vi "ABB Test Locked Rotor.vi"() -> ()   [LabVIEW 2017]
uses:
  Temp error msg.ctl
  ABB global.vi
panel:
  in  "Temp error":T1="Error: Temperature measurement "
  out "Auto Readings":cluster{"%":dbl[], "Recorded":bool[]}
  in  "Simulate I":dbl(slide)
  out "Readings":string[][](table)
  out "In Range?":bool[](array[boolean])
  out "saved Readings":dbl[][](array[numeric])
  out "% rated current":dbl format="%.1f"
  out "Rated Current":dbl
  out "Serial number":string
  out "W.O number":string
  out "Power":string[][](table)
  out "Current & Voltage":string[][](table)
  out "Norma 5000 Error":string
  in  "Record":bool
  out "Readings":string[][](table)
  in  "View":enum16{"Graph", "Readings"}(ring)
  out "Number readings":i32
  out "Status":enum16{"Stopped", "Running"}(ring)
  out "Timedate":string
  in  "End test":bool
  in  "Start":bool
  in  "Read Mode":enum16{"Auto", "Manual"}(ring)
  in  "Exit":bool
  out "Current vs Voltage":T2(graph)
  # "Locked Rotor Test"
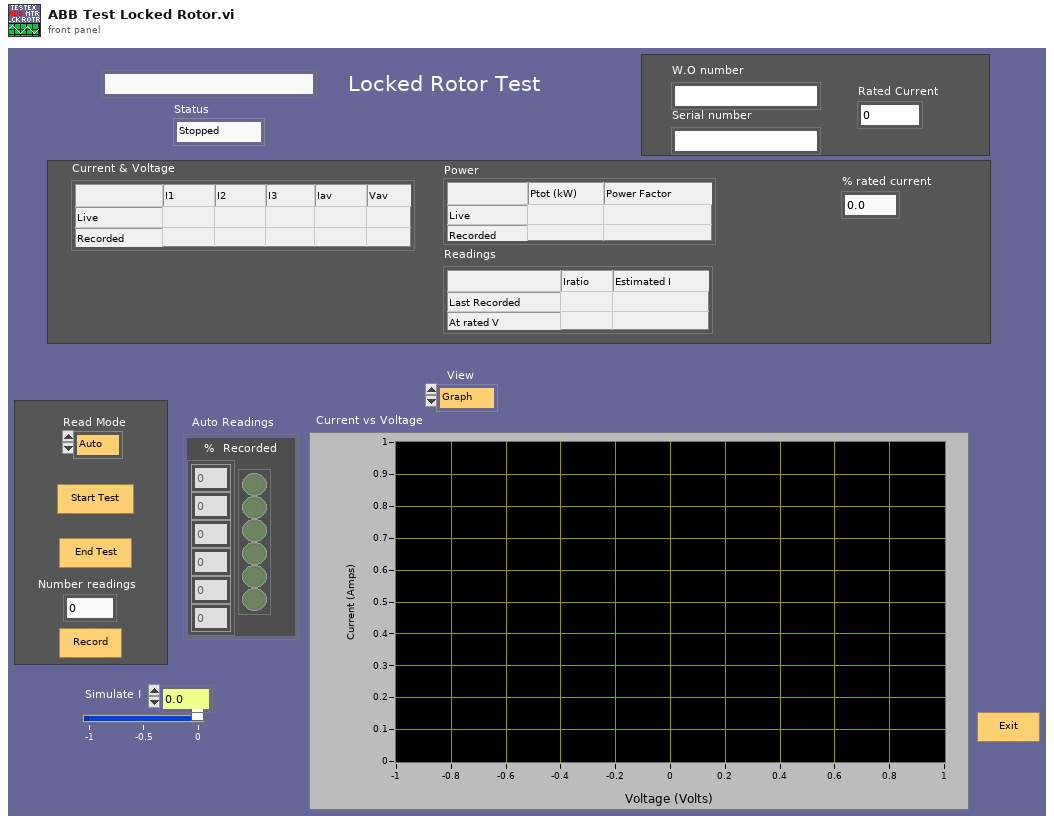
[diagram p1: front panel]
types:
  T1 = typedef "Temp error msg.ctl" = string
  T2 = cluster{"Sorted 2D Array":dbl[], "Sorted 2D Array":dbl[]}
  T3 = cluster{"Voltage":dbl, "Power":dbl, "Current":dbl, "PF":dbl}
  T4 = cluster{"VT Primary":dbl, "VT Secondary":dbl, "CT  Primary":dbl, "CT Secondary":dbl, "Current Shunt":enum16{"Internal", "External"}, "Avg interval":dbl}
  T5 = cluster{"VT Primary":dbl, "VT Secondary":dbl, "CT  Primary":dbl, "CT Secondary":dbl, "Current Shunt":enum16{"Internal", "External"}, "Averaging interval (secs)":dbl}
  T6 = cluster{"Visa sesssion":refnum<visa-resource-name>, "error":errorcluster}
  T7 = cluster{"Simulate Norma":bool, "Norma 5000 Address":u8, "WebDaq IP Address":string, "Simulate cDAQ":bool}
  T8 = cluster{"Number Values":i32, "Tolerance":dbl, "Value (ratio) ":dbl[], "Hold time (sec)":dbl}
  T9 = cluster{"V":dbl, "A":dbl, "W":dbl, "VA":dbl, "VAr":dbl, "Pf":dbl}
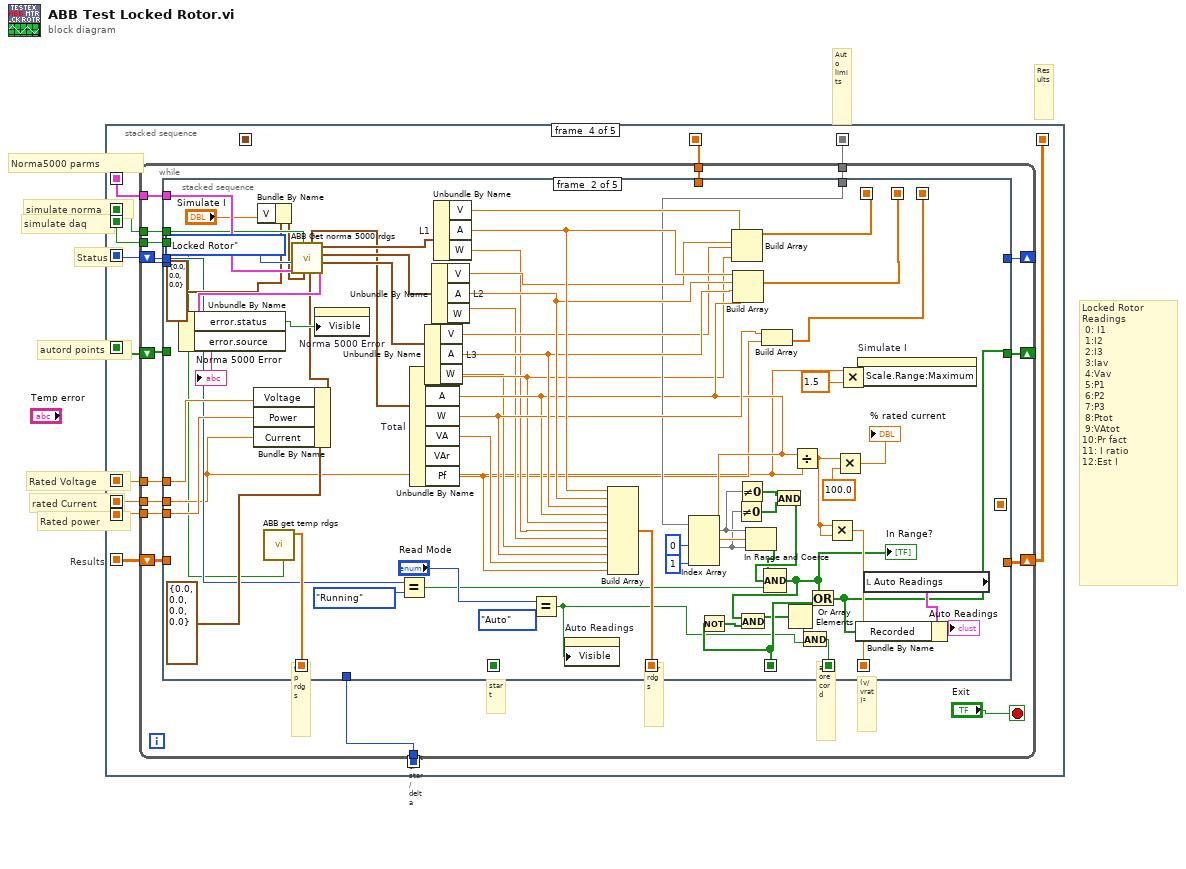
[diagram p0: block diagram]
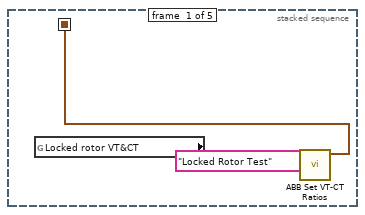
[diagram p2: hidden frame]
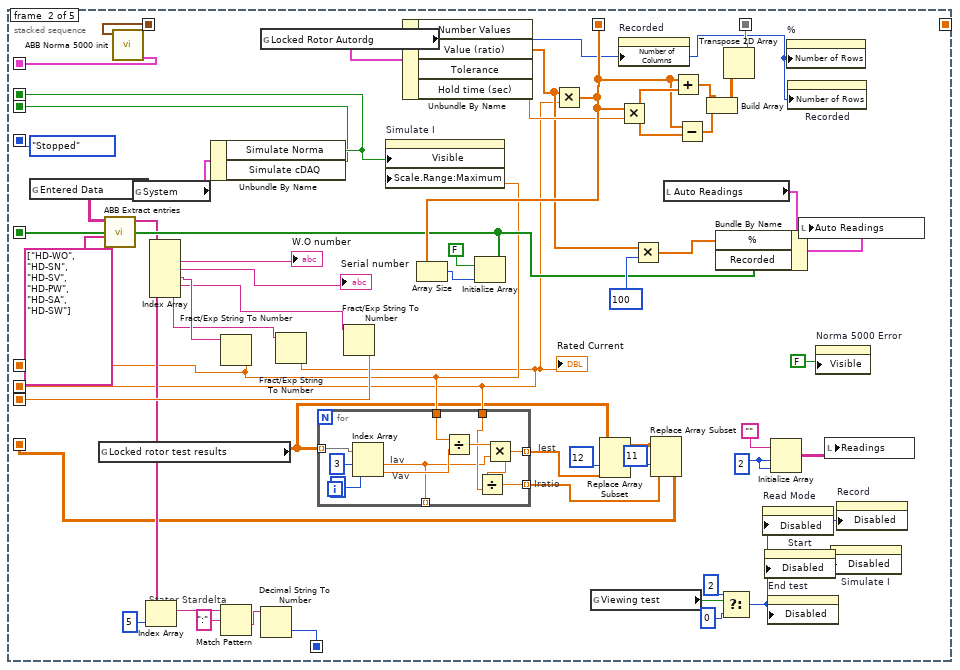
[diagram p3: hidden frame]
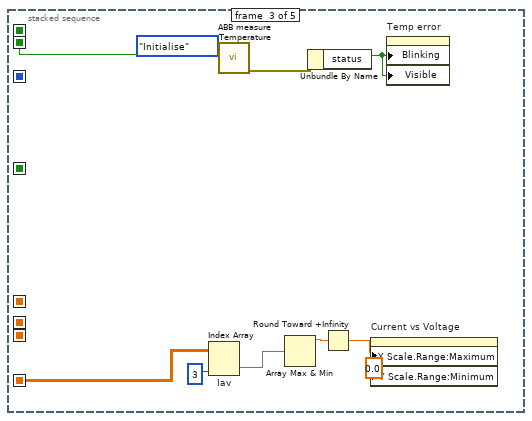
[diagram p4: hidden frame]
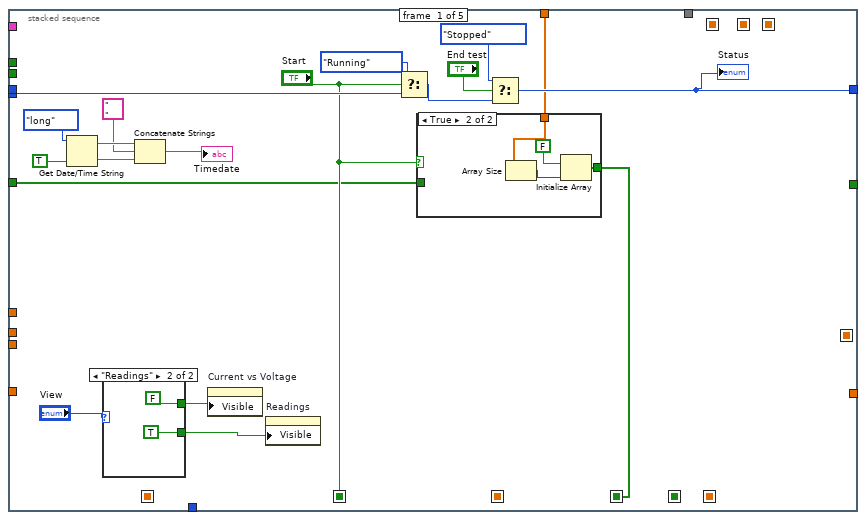
[diagram p5: hidden frame]
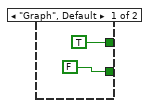
[diagram p7: hidden frame]
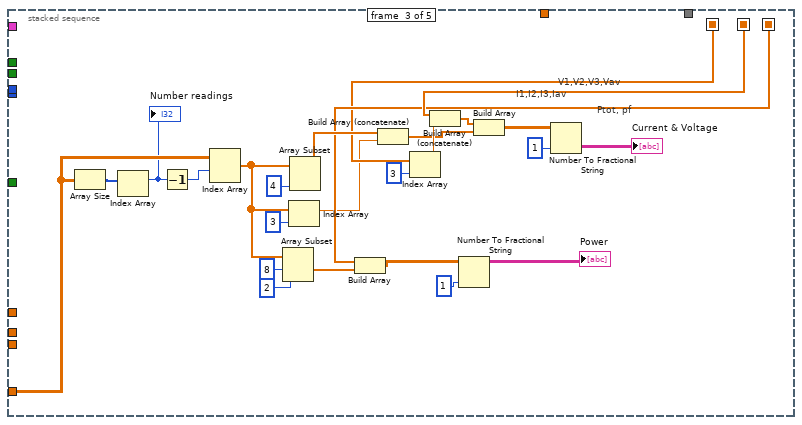
[diagram p8: hidden frame]
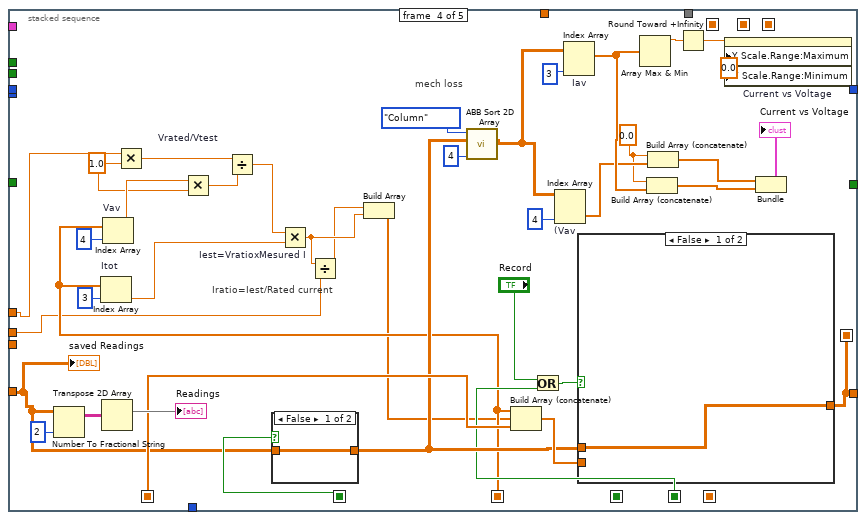
[diagram p9: hidden frame]
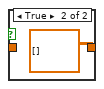
[diagram p10: hidden frame]
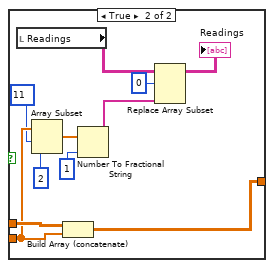
[diagram p11: hidden frame]
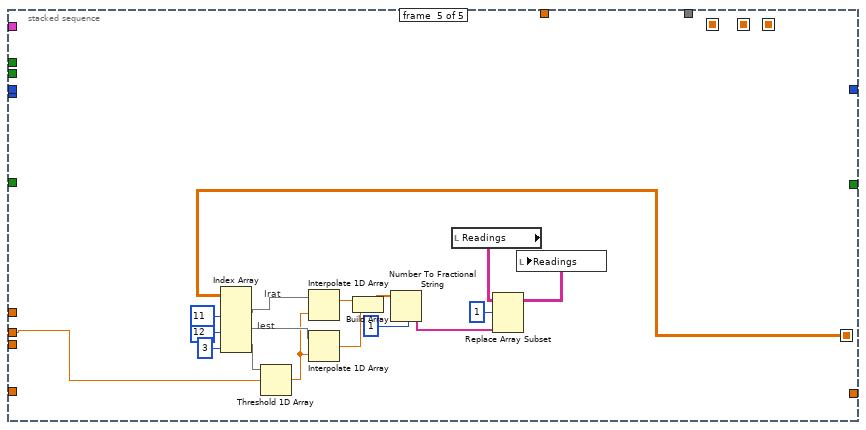
[diagram p12: hidden frame]
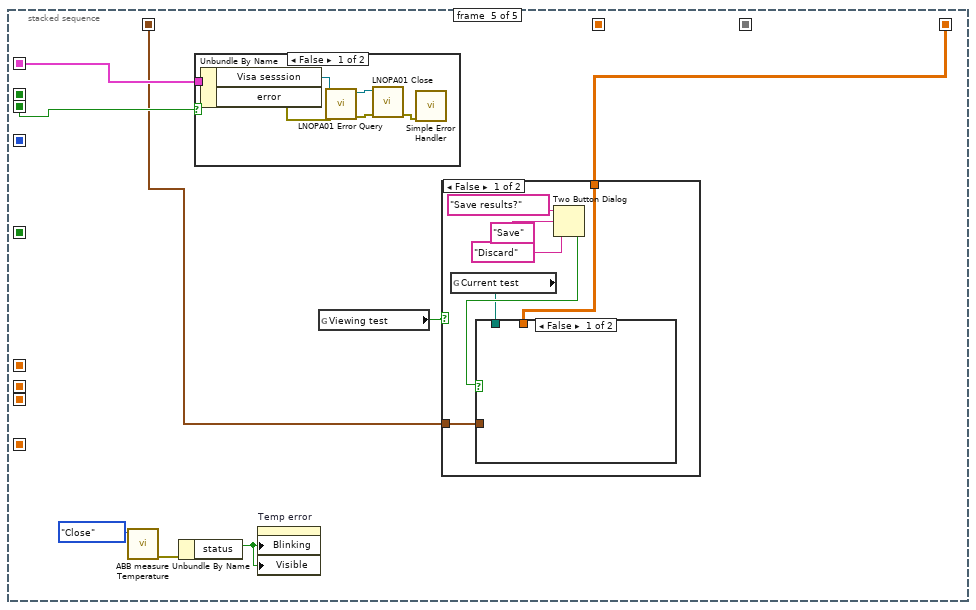
[diagram p13: hidden frame]
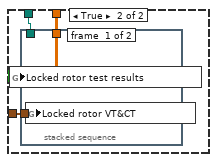
[diagram p14: hidden frame]
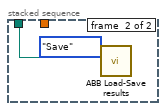
[diagram p15: hidden frame]
diagram:
  # "Results"
  # "stator star/delta"
  # "simulate daq"
  # "Results"
  # "Rated power"
  # "Rated Voltage"
  # "Locked Rotor\nReadings\n 0: I1\n 1:I2\n 2:I3\n 3:Iav\n 4:Vav\n 5:P1\n 6:P2\n 7:P3\n 8:Ptot\n 9:VAtot\n10:Pr fact\n11: I ratio\n12:Est I"
  # "autord points"
  # "Auto limits"
  # "rated Current"
  # "simulate norma"
  # "Norma5000 parms"
  # "Status"
  n1 = stacked-sequence {
    seq-local: [_ enum16{"Stopped", "Running"}."Stopped" ("Status") _ _ _] -> [_ _ _ w90 _]
    seq-local: [_ w56 _ _ _] -> [_ _ _ w89 w306]
    seq-local: [_ w42 _ _ _] -> [_ _ _ w88 w305]
    seq-local: [_ w11 _ _ _] -> [_ _ _ w87 _]
    seq-local: [_ w4 _ _ _] -> [_ _ w72 w86 _]
    seq-local: [_ w24 _ _ _] -> [_ _ _ w85 _]
    seq-local: [_ w48 _ _ _] -> [_ _ _ w83 _]
    seq-local: [_ w46 _ _ _] -> [_ _ _ w84 _]
    seq-local: [_ w12 _ _ _] -> [_ _ _ w82 _]
    seq-local: [_ w43 _ _ _] -> [_ _ _ w81 _]
    seq-local: [_ _ _ w80 _] -> [_ _ _ _ w303]
    seq-local: [_ w30 _ _ _] -> [_ _ w71 w78 _]
    seq-local: [_ w17 _ _ _] -> [_ _ _ w79 _]
    seq-local: [w1 _ _ _ _] -> [_ w13 _ _ w302]
    frame #0 {
      n2 = global read "ABB global.vi" "Locked rotor VT&CT"() -> (w3:T4)
      n3 = call "ABB Set VT-CT Ratios.vi"("Test name"="Locked Rotor Test", "VT and CT Ratios"=w3) -> ("VT and CT Ratios out"=w1:T5)  [unwired: 9 in]
    }
    frame #1 {
      w14 = 2
      # "Iratio"
      # "Iest"
      # "Stator Stardelta"
      n4 = global read "ABB global.vi" "Entered Data"() -> (w41:string[][])
      n5 = global read "ABB global.vi" "Locked rotor test results"() -> (w10:dbl[][])
      n6 = call "ABB Extract entries.vi"("Entry IDs"=string[] ["HD-WO", "HD-SN", "HD-SV", "HD-PW", "HD-SA", "HD-SW"], "Entry table in"=w41) -> ("Selected Entries"=w18:string[])  [unwired: 9 in]
      n7 = call "ABB Norma 5000 init.vi"("VT and CT Ratios"=w13) -> ("norma 5000 parms out"=w56:T6)  [unwired: 10 in]
      n8 = global read "ABB global.vi" "System"() -> (w55:T7)
      n9 = Index Array(array=w18, index=5) -> (element=w21:string)
      n10 = Index Array(array=w18) -> (element #1=→"W.O number":string, element #2=→"Serial number":string, element #3=w37:string, element #4=w36:string, element #5=w35:string)  [unwired: 5 in]
      n11 = Unbundle By Name(w55) -> ("Simulate Norma"=w42:bool, "Simulate cDAQ"=w30:bool)
      n12 = Fract/Exp String To Number(string=w37) -> (number=w12:dbl)  [unwired: 3 in, 1 out]
      n13 = Match Pattern(string=w21, regular expression=":") -> (after substring=w19:string)  [unwired: 1 in, 3 out]
      n14 = global read "ABB global.vi" "Locked Rotor Autordg"() -> (w45:T8)
      n15 = Decimal String To Number(string=w19) -> (number=w17:i32)  [unwired: 2 in, 1 out]
      n16 = Fract/Exp String To Number(string=w35) -> (number=w11:dbl)  [unwired: 3 in, 1 out]
      "Rated Current" <- w11
      n17 = for {
        tunnel: w10 -> [w67] mode=indexing
        tunnel: w12 -> [w63]
        tunnel: w11 -> [w61]
        tunnel: [w60] -> w8 mode=indexing
        tunnel: [w59] -> w7 mode=indexing
        tunnel: [w58] -> _ mode=indexing
        # "Vav"
        # "Iav"
        n18 = Index Array(array=w67, index #1=3 ("index"), index #2=4) -> (element #1=w58:dbl, element #2=w64:dbl)
        n19 = Divide(x=w63, y=w64) -> (x/y=w62:dbl)
        n20 = Multiply(x=w62, y=w58) -> (x*y=w60:dbl)
        n21 = Divide(x=w60, y=w61) -> (x/y=w59:dbl)
      }
      n22 = Fract/Exp String To Number(string=w36) -> (number=w43:dbl)  [unwired: 3 in, 1 out]
      n23 = property on="Simulate I" class="Slide (strict)"("Visible"=w42, "Scale.Range:Maximum"=w12) -> ()  [unwired: 2 in, 2 out]
      n24 = Unbundle By Name(w45) -> ("Number Values"=w23:i32, "Value (ratio)"=w29:dbl[], "Tolerance"=w44:dbl)  [unwired: 1 out]
      n25 = Multiply(x=w29, y=w11) -> (x*y=w46:dbl[])
      n26 = Array Size(array=w46) -> (size(s)=w53:i32)
      n27 = Initialize Array(FALSE, w53) -> (w24:bool[])
      n28 = global read "ABB global.vi" "Viewing test"() -> (w34:bool)
      n29 = Replace Array Subset(array=w10, new element=w8, index (col)=12 ("index (row)")) -> (w9:dbl[][])  [unwired: 1 in]
      n30 = property on="Recorded" class="Arr (strict)"("Number of Columns"=w23) -> ()  [unwired: 2 in, 2 out]
      n31 = Multiply(x=w46, y=w44) -> (x*y=w50:dbl[])
      n32 = Multiply(x=w29, y=100 ("Numeric")) -> (x*y=w25:dbl[])
      n33 = Replace Array Subset(array=w9, new element=w7, index (col)=11 ("index (row)")) -> (w4:dbl[][])  [unwired: 1 in]
      n34 = local read "Auto Readings"() -> (w27:cluster{"%":dbl[], "Recorded":bool[]})
      n35 = Add(x=w46, y=w50) -> (x+y=w51:dbl[])
      n36 = Subtract(x=w46, y=w50) -> (x-y=w47:dbl[])
      n37 = Build Array(w51, w47) -> (w49:dbl[][])
      n38 = Bundle By Name(cluster=w27, "%"=w25, "Recorded"=w24) -> (w26:cluster{"%":dbl[], "Recorded":bool[]})
      n39 = Select(t=2, s=w34, f=0) -> (s? t:f=w31:i32)
      n40 = Transpose 2D Array(2D array=w49) -> (transposed array=w48:dbl[][])
      n41 = property on="Read Mode" class="Enum (strict)"("Disabled"=w31) -> ()  [unwired: 2 in, 2 out]
      n42 = property on="Start" class="Bool"("Disabled"=w31) -> ()  [unwired: 2 in, 2 out]
      n43 = property on="End test" class="Bool"("Disabled"=w31) -> ()  [unwired: 2 in, 2 out]
      n44 = Initialize Array("", w14, w14) -> (w16:string[][])
      n45 = property on="%" class="Arr (strict)"("Number of Rows"=w23) -> ()  [unwired: 2 in, 2 out]
      n46 = property on="Recorded" class="Arr (strict)"("Number of Rows"=w23) -> ()  [unwired: 2 in, 2 out]
      n47 = local write "Auto Readings"(w26) -> ()
      n48 = property on="Norma 5000 Error" class="Str"("Visible"=FALSE) -> ()  [unwired: 2 in, 2 out]
      n49 = local write "Readings"(w16) -> ()
      n50 = property on="Simulate I" class="Slide (strict)"("Disabled"=w31) -> ()  [unwired: 2 in, 2 out]
      n51 = property on="Record" class="Bool"("Disabled"=w31) -> ()  [unwired: 2 in, 2 out]
    }
    frame #2 {
      n52 = Index Array "Iav"(array=w72, index (col)=3 ("disabled index (col)")) -> (element=w74:dbl[])  [unwired: 1 in]
      n53 = call "ABB measure Temperature.vi"("Simulate"=w71, "Mode"=enum16{"Initialise", "Read", "Close"}."Initialise") -> ("error out"=w69:errorcluster)  [unwired: 7 in, 2 out]
      n54 = Array Max & Min(array=w74) -> (max value=w77:dbl)  [unwired: 3 out]
      n55 = Unbundle By Name(w69) -> ("status"=w68:bool)
      n56 = Round Toward +Infinity(x=w77) -> (ceil(x): smallest int >= x=w73:dbl)
      n57 = property on="Current vs Voltage" class="XYGraph (strict)"("Y Scale.Range:Maximum"=w73, "Y Scale.Range:Minimum"=0.0) -> ()  [unwired: 2 in, 2 out]
      n58 = property on="Temp error" class="Str (strict)"("Blinking"=w68, "Visible"=w68) -> ()  [unwired: 2 in, 2 out]
    }
    frame #3 {
      n59 = while {
        shift-right: [w105] -> _
        shift-left: w90 -> [w93]
        tunnel: w89 -> [w104]
        tunnel: w88 -> [w103]
        tunnel: w87 -> [w102]
        shift-right: [w100] -> w80
        shift-left: w86 -> [w101]
        shift-right: [w99] -> _
        shift-left: w85 -> [w98]
        tunnel: w84 -> [w97]
        tunnel: w83 -> [w96]
        tunnel: w82 -> [w95]
        tunnel: w81 -> [w94]
        tunnel: w79 -> [w92]
        tunnel: w78 -> [w91]
        stop <- "Exit" stop-if-true
        # "autorecord"
        # "(v/vrat)²"
        # "temp rdgs"
        # "pwr rdgs"
        # "start"
        n60 = stacked-sequence {
          seq-local: ["Start" _ _ _ _] -> [_ _ _ w267 _]
          seq-local: [_ w184 _ _ _] -> [_ _ _ w250 _]
          seq-local: [_ w183 _ _ _] -> [_ _ _ w261 _]
          seq-local: [_ w181 _ _ _] -> [_ _ _ _ _]
          seq-local: [w107 _ _ _ _] -> [_ w177 _ _ _]
          seq-local: [_ w175 _ _ _] -> [_ _ _ w253 _]
          seq-local: [_ w172 _ _ _] -> [_ _ w207 _ _]
          seq-local: [_ w171 _ _ _] -> [_ _ w221 _ _]
          seq-local: [_ w170 _ _ _] -> [_ _ w213 _ _]
          seq-local: [_ _ _ w231 _] -> [_ _ _ _ w298]
          tunnel: w93 -> [w119 _ _ _ _]
          tunnel: [w114 _ _ _ _] -> w105
          tunnel: w104 -> [_ w202 _ _ _]
          tunnel: w103 -> [_ w194 _ _ _]
          tunnel: w102 -> [_ w151 _ w229 w293]
          tunnel: w101 -> [_ _ w226 w233 _]
          tunnel: [_ _ _ w231 _] -> w100
          tunnel: [_ w145 _ _ _] -> w99
          tunnel: w98 -> [w109 _ _ _ _]
          tunnel: w97 -> [w108 _ _ _ _]
          tunnel: w96 -> [_ w180 _ _ _]
          tunnel: w95 -> [_ w161 _ w239 _]
          tunnel: w94 -> [_ w160 _ _ _]
          tunnel: w93 -> [_ w154 _ _ _]
          tunnel: w92 -> [_ _ _ _ _]
          tunnel: w91 -> [_ w135 _ _ _]
          frame #0 {
            n61 = Get Date/Time String(date format (0)=enum16{"short", "long", "abbreviated"}."long", want seconds? (F)=TRUE) -> (date string=w123:string, time string=w122:string)  [unwired: 1 in]
            n62 = case shown="\"Readings\"" "View" {
              tunnel: [TRUE FALSE] -> w112
              tunnel: [FALSE TRUE] -> w111
              frame "Graph", Default {
              }
              frame "Readings" {
              }
            }
            n63 = Concatenate Strings(w123, "   ", w122) -> (→"Timedate":string)
            n64 = property on="Current vs Voltage" class="XYGraph (strict)"("Visible"=w112) -> ()  [unwired: 2 in, 2 out]
            n65 = property on="Readings" class="Tbl (strict)"("Visible"=w111) -> ()  [unwired: 2 in, 2 out]
            n66 = Select(t=enum16{"Stopped", "Running"}."Running", s="Start", f=w119) -> (s? t:f=w117:enum16{"Stopped", "Running"})
            n67 = case shown="True" "Start" {
              tunnel: w108 -> [_ w130]
              tunnel: [w126 w127] -> w107
              tunnel: w109 -> [w126 _]
              frame False {
              }
              frame True {
                n68 = Array Size(array=w130) -> (size(s)=w129:i32)
                n69 = Initialize Array(FALSE, w129) -> (w127:bool[])
              }
            }
            n70 = Select(t=enum16{"Stopped", "Running"}."Stopped", s="End test", f=w117) -> (s? t:f=w114:enum16{"Stopped", "Running"})
            "Status" <- w114
          }
          frame #1 {
            n71 = Bundle By Name(cluster=T3 {"Voltage"=0.0, "Power"=0.0, "Current"=0.0, "PF"=0.0} ("Rated"), "Voltage"=w161, "Power"=w160, "Current"=w151) -> (w159:T3)
            n72 = Bundle By Name(cluster=cluster{"V":dbl, "A":dbl, "pwr factor":dbl} {"V"=0.0, "A"=0.0, "pwr factor"=0.0} ("Simulation rdgs"), "V"="Simulate I") -> (w156:cluster{"V":dbl, "A":dbl, "pwr factor":dbl})
            n73 = call "ABB get temp rdgs.vi"("Sim daq"=w135) -> ("Category rdgs"=w183:dbl[])  [unwired: 7 in, 3 out]
            n74 = call "ABB Get norma 5000 rdgs.vi"("Rated"=w159, "Simulation rdgs"=w156, "simulate"=w194, "norma 5000 parms in"=w202, "Simulate Mode"=enum16{"No load", "Locked Rotor"}."Locked Rotor") -> ("norma 5000 parms out"=w196:T6, "L 3"=w197:T9, "L 2"=w198:T9, "L1"=w199:T9, "Total"=w195:T9)  [unwired: 2 in]
            n75 = Unbundle By Name(w196) -> ("error.status"=w201:bool, "error.source"=→"Norma 5000 Error":string)
            n76 = property on="Norma 5000 Error" class="Str"("Visible"=w201) -> ()  [unwired: 2 in, 2 out]
            n77 = Equal?(x=w154, y=enum16{"Stopped", "Running"}."Running") -> (x = y?=w152:bool)
            n78 = Unbundle By Name "Total"(w195) -> ("V"=w168:dbl, "A"=w169:dbl, "W"=w185:dbl, "VA"=w164:dbl, "Pf"=w163:dbl)  [unwired: 1 out]
            n79 = Unbundle By Name "L3"(w197) -> ("V"=w186:dbl, "A"=w189:dbl, "W"=w165:dbl)
            n80 = Unbundle By Name "L2"(w198) -> ("V"=w187:dbl, "A"=w190:dbl, "W"=w166:dbl)
            n81 = Unbundle By Name "L1"(w199) -> ("V"=w188:dbl, "A"=w191:dbl, "W"=w167:dbl)
            n82 = Equal?(x="Read Mode", y=enum16{"Auto", "Manual"}."Auto") -> (x = y?=w148:bool)
            n83 = property on="Auto Readings" class="Clust (strict)"("Visible"=w148) -> ()  [unwired: 2 in, 2 out]
            n84 = Build Array(w191, w190, w189, w169, w168, w167, w166, w165, w185, w164, w163) -> (w184:dbl[])
            n85 = Index Array(array=w180, index (col) #1=0 ("disabled index (col)"), index (col) #2=1 ("index (col)")) -> (element #1=w142:dbl[], element #2=w141:dbl[])  [unwired: 2 in]
            n86 = Not(x=w177) -> (.not. x?=w139:bool[])
            n87 = Build Array(w188, w187, w186, w168) -> (w172:dbl[])
            n88 = Build Array(w191, w190, w189, w169) -> (w171:dbl[])
            n89 = Not Equal To 0?(x=w141) -> (x != 0?=w143:bool[])
            n90 = Not Equal To 0?(x=w142) -> (x != 0?=w144:bool[])
            n91 = In Range and Coerce(upper limit=w142, x=w169, lower limit=w141) -> (In Range?=w138:bool[])  [unwired: 1 out]
            n92 = Build Array(w185, w163) -> (w170:dbl[])
            n93 = And(x=w144, y=w143) -> (x .and. y?=w140:bool[])
            n94 = Compound Arithmetic op=AND(w138, w140, w152) -> (w136:bool[])
            "In Range?" <- w136
            n95 = And(x=w136, y=w139) -> (x .and. y?=w137:bool[])
            n96 = Or Array Elements(Boolean array=w137) -> (logical OR=w176:bool)
            n97 = Divide(x=w169, y=w151) -> (x/y=w182:dbl)
            n98 = And(x=w176, y=w148) -> (x .and. y?=w175:bool)
            n99 = Or(x=w136, y=w177) -> (x .or. y?=w145:bool[])
            n100 = Multiply(x=w182, y=w182) -> (x*y=w181:dbl)
            n101 = Multiply(x=w182, y=100.0) -> (x*y=→"% rated current":dbl)
            n102 = Multiply(x=w151, y=1.5) -> (x*y=w149:dbl)
            n103 = property on="Simulate I" class="Slide (strict)"("Scale.Range:Maximum"=w149) -> ()  [unwired: 2 in, 2 out]
            n104 = local read "Auto Readings"() -> (w147:cluster{"%":dbl[], "Recorded":bool[]})
            n105 = Bundle By Name(cluster=w147, "Recorded"=w145) -> (→"Auto Readings":cluster{"%":dbl[], "Recorded":bool[]})
          }
          frame #2 {
            # "I1,I2,I3,Iav"
            # "V1,V2,V3,Vav"
            # "Ptot, pf"
            n106 = Array Size(array=w226) -> (size(s)=w227:i32[])
            n107 = Index Array(array=w227) -> (element=w210:i32)  [unwired: 1 in]
            "Number readings" <- w210
            n108 = Decrement(x=w210) -> (x-1=w225:i32)
            n109 = Index Array(array=w226, index (row)=w225) -> (element=w211:dbl[])  [unwired: 1 in]
            n110 = Array Subset(array=w211, index=8, length=2) -> (w214:dbl[])
            n111 = Index Array(array=w211, index=3) -> (element=w203:dbl)
            n112 = Array Subset(array=w211, length=4) -> (w220:dbl[])  [unwired: 1 in]
            n113 = Build Array(w213, w214) -> (w215:dbl[][])
            n114 = Build Array (concatenate)(w220, w203) -> (w205:dbl[])
            n115 = Index Array(array=w207, index=3) -> (element=w206:dbl)
            n116 = Build Array (concatenate)(w221, w206) -> (w208:dbl[])
            n117 = Number To Fractional String(number=w215, precision (6)=i16 1) -> (F-format string=→"Power":string[][])  [unwired: 2 in]
            n118 = Build Array(w208, w205) -> (w219:dbl[][])
            n119 = Number To Fractional String(number=w219, precision (6)=i16 1) -> (F-format string=→"Current & Voltage":string[][])  [unwired: 2 in]
          }
          frame #3 {
            w232 = 1.0 ("y")
            w234 = 0.0
            # "Iratio=Iest/Rated current"
            # "mech loss"
            n120 = Number To Fractional String(number=w233, precision (6)=i16 2) -> (F-format string=w266:string[][])  [unwired: 2 in]
            n121 = Index Array "Itot"(array=w250, index=3) -> (element=w238:dbl)
            n122 = Transpose 2D Array(2D array=w266) -> (transposed array=→"Readings":string[][])
            n123 = Index Array "Vav"(array=w250, index=4) -> (element=w242:dbl)
            n124 = Multiply(x=w239, y=w232) -> (x*y=w240:dbl)
            n125 = Multiply(x=w242, y=w232) -> (x*y=w241:dbl)
            n126 = Divide "Vrated/Vtest"(x=w240, y=w241) -> (x/y=w244:dbl)
            n127 = case shown="False" w267 {
              tunnel: w233 -> [w268 _]
              tunnel: [w268 dbl[][] []] -> w255
              frame False {
              }
              frame True {
              }
            }
            n128 = Multiply "Iest=VratioxMesured I"(x=w244, y=w238) -> (x*y=w230:dbl)
            n129 = Divide(x=w230, y=w229) -> (x/y=w228:dbl)
            n130 = Build Array(w228, w230) -> (w243:dbl[])
            n131 = call "ABB Sort 2D Array.vi"("Column/Row to Sort By"=u32 4, "Unsorted 2D Array"=w255, "Sort by"=enum16{"Column", "Row"}."Column") -> ("Sorted 2D Array"=w248:dbl[][])  [unwired: 4 in]
            n132 = Build Array (concatenate)(w250, w243, w261) -> (w262:dbl[])
            n133 = Or(x="Record", y=w253) -> (x .or. y?=w254:bool)
            n134 = Index Array "(Vav"(array=w248, index (col)=4 ("disabled index (col)")) -> (element=w245:dbl[])  [unwired: 1 in]
            n135 = Index Array "Iav"(array=w248, index (col)=3 ("disabled index (col)")) -> (element=w247:dbl[])  [unwired: 1 in]
            n136 = case shown="False" w254 {
              tunnel: w255 -> [w270 w281]
              tunnel: [w270 w280] -> w231
              tunnel: w262 -> [_ w275]
              frame False {
              }
              frame True {
                n137 = local read "Readings"() -> (w278:string[][])
                n138 = Array Subset(array=w275, index=11, length=2) -> (w272:dbl[])
                n139 = Build Array (concatenate)(w281, w275) -> (w280:dbl[][])
                n140 = Number To Fractional String(number=w272, precision (6)=i16 1) -> (F-format string=w271:string[])  [unwired: 2 in]
                n141 = Replace Array Subset(array=w278, new element=w271, index (row)=0) -> (→"Readings":string[][])  [unwired: 1 in]
              }
            }
            n142 = Array Max & Min(array=w247) -> (max value=w258:dbl)  [unwired: 3 out]
            n143 = Build Array (concatenate)(w234, w247) -> (w235:dbl[])
            n144 = Build Array (concatenate)(w234, w245) -> (w236:dbl[])
            n145 = Round Toward +Infinity(x=w258) -> (ceil(x): smallest int >= x=w246:dbl)
            n146 = property on="Current vs Voltage" class="XYGraph (strict)"("Y Scale.Range:Maximum"=w246, "Y Scale.Range:Minimum"=0.0) -> ()  [unwired: 2 in, 2 out]
            n147 = Bundle(w236, w235) -> (→"Current vs Voltage":cluster{dbl[], dbl[]})  [unwired: 1 in]
            "saved Readings" <- w233
          }
          frame #4 {
            # "Iest"
            # "Irat"
            n148 = Index Array(array=w298, index (col) #1=11 ("disabled index (col)"), index (col) #2=12 ("index (col)"), index (col) #3=3 ("index (col)")) -> (element #1=w292:dbl[], element #2=w291:dbl[], element #3=w294:dbl[])  [unwired: 3 in]
            n149 = Threshold 1D Array(2:w293, 3:w294) -> (0:w290:dbl)  [unwired: 1 in]
            n150 = Interpolate 1D Array(1:w290, 2:w292) -> (0:w285:dbl)
            n151 = Interpolate 1D Array(1:w290, 2:w291) -> (0:w284:dbl)
            n152 = Build Array(w285, w284) -> (w283:dbl[])
            n153 = Number To Fractional String(number=w283, precision (6)=i16 1) -> (F-format string=w282:string[])  [unwired: 2 in]
            n154 = local read "Readings"() -> (w288:string[][])
            n155 = Replace Array Subset(array=w288, new element=w282, index (row)=1) -> (w287:string[][])  [unwired: 1 in]
            n156 = local write "Readings"(w287) -> ()
          }
        }
      }
    }
    frame #4 {
      n157 = call "ABB measure Temperature.vi"("Mode"=enum16{"Initialise", "Read", "Close"}."Close") -> ("error out"=w299:errorcluster)  [unwired: 8 in, 2 out]
      n158 = Unbundle By Name(w299) -> ("status"=w300:bool)
      n159 = case shown="False" w305 {
        tunnel: w306 -> [w323 _]
        frame False {
          n160 = Unbundle By Name(w323) -> ("Visa sesssion"=w322:refnum<visa-resource-name>, "error"=w321:errorcluster)
          n161 = call "LNOPA01 Error Query.vi"("error in (no error)"=w321, "VISA session"=w322) -> ("error out"=w324:errorcluster, "dup VISA session"=w325:refnum<visa-resource-name>)  [unwired: 6 in, 2 out]
          n162 = call "LNOPA01 Close.vi"("error in (no error)"=w324, "VISA session"=w325) -> ("error out"=w326:errorcluster)  [unwired: 9 in]
          n163 = call <vilib>:"Simple Error Handler.vi"("error in (no error)"=w326) -> ()  [unwired: 4 in, 5 out]
        }
        frame True {
        }
      }
      n164 = property on="Temp error" class="Str (strict)"("Blinking"=w300, "Visible"=w300) -> ()  [unwired: 2 in, 2 out]
      n165 = global read "ABB global.vi" "Viewing test"() -> (w304:bool)
      n166 = case shown="False" w304 {
        tunnel: w303 -> [w311 _]
        tunnel: w302 -> [w307 _]
        frame False {
          n167 = global read "ABB global.vi" "Current test"() -> (w310:path)
          n168 = Two Button Dialog(message="Save results?", 1:"Discard" ("F button name (\"Cancel\")"), 2:"Save" ("T button name (\"OK\")")) -> (T button?=w312:bool)
          n169 = case shown="False" w312 {
            tunnel: w311 -> [_ w316]
            tunnel: w310 -> [_ w315]
            tunnel: w307 -> [_ w314]
            frame False {
            }
            frame True {
              n170 = stacked-sequence {
                tunnel: w316 -> [w318 _]
                tunnel: w315 -> [_ w319]
                tunnel: w314 -> [w317 _]
                frame #0 {
                  n171 = global write "ABB global.vi" "Locked rotor test results"(w318) -> ()
                  n172 = global write "ABB global.vi" "Locked rotor VT&CT"(w317) -> ()
                }
                frame #1 {
                  n173 = call "ABB Load-Save results.vi"("Path"=w319, "Mode"=enum16{"LOAD", "Save"}."Save") -> ()  [unwired: 10 in]
                }
              }
            }
          }
        }
        frame True {
        }
      }
    }
  }
